vi "0_MNIST(Train).vi"() -> ()   [LabVIEW 2020]
uses:
  <vilib>/Ngene/Deep Learning Toolkit/Toolkit/NN_Train/Controls/NN_Train_Params.ctl
  <vilib>/Ngene/Deep Learning Toolkit/Toolkit/NN_Train/Controls/NN_Train_Optimizer.ctl
  <vilib>/Ngene/Deep Learning Toolkit/Toolkit/NN_Train/Controls/NN_Train_Data_Sampling.ctl
  Controls/Img_GrayScale.ctl
  <vilib>/Ngene/Deep Learning Toolkit/Toolkit/NN_Train/Controls/NN_Train_Session_Data.ctl
  <vilib>/Ngene/Deep Learning Toolkit/Toolkit/NN_Train/Controls/NN_LR_Policy_Cfg.ctl
  <vilib>/Ngene/Deep Learning Toolkit/Toolkit/NN_Train/Controls/NN_LR_Policy_Type.ctl
  <vilib>/Ngene/Deep Learning Toolkit/Toolkit/NN_Network/Controls/NN_Device.ctl
  <vilib>/Ngene/Deep Learning Toolkit/Toolkit/NN_Layers/Layers/Pool/Controls/NN_Layer_Config(Pool).ctl
  <vilib>/Ngene/Deep Learning Toolkit/Toolkit/NN_Data/API/NN_Dims(V,H).ctl
  <vilib>/Ngene/Deep Learning Toolkit/Toolkit/NN_Layers/Layers/Conv2D/Controls/NN_Conv2D_Padding_Type.ctl
  <vilib>/Ngene/Deep Learning Toolkit/Toolkit/NN_Layers/Layers/Conv2D/Controls/NN_Layer_Config(Conv2D).ctl
  <vilib>/Ngene/Deep Learning Toolkit/Toolkit/NN_Layers/Layers/Conv2D/Controls/NN_Layer_Params(Conv2D).ctl
  <vilib>/Ngene/Deep Learning Toolkit/Toolkit/NN_Layers/Layers/BatchNorm/Controls/NN_BN_Params.ctl
  <vilib>/Ngene/Deep Learning Toolkit/Toolkit/NN_Activations/Controls/NN_Activation_Type.ctl
  <vilib>/Ngene/Deep Learning Toolkit/Toolkit/NN_Layers/Controls/NN_Layer_Init_Params.ctl
  <vilib>/Ngene/Deep Learning Toolkit/Toolkit/NN_Layers/Controls/NN_Layer_Weight_Init_Type.ctl
  <vilib>/Ngene/Deep Learning Toolkit/Toolkit/NN_Layers/Layers/FC/Controls/NN_Layer_Config(FC).ctl
  <vilib>/Ngene/Deep Learning Toolkit/Toolkit/NN_Network/Controls/NN_Save_Before_Destroy_Options.ctl
  <vilib>/Ngene/Deep Learning Toolkit/Toolkit/NN_Layers/Layers/Input/Controls/NN_Layer_Config(Input3D).ctl
  <vilib>/Ngene/Deep Learning Toolkit/Toolkit/NN_Data/API/NN_Dims(C,H,W).ctl
  <vilib>/Ngene/Deep Learning Toolkit/Toolkit/NN_Data/Controls/NN_Data_type.ctl
  <vilib>/Ngene/Deep Learning Toolkit/Toolkit/NN_Layers/Layers/Input/NN_Layer_Create(Input3D).vi
  <vilib>/Ngene/Deep Learning Toolkit/Toolkit/NN_Layers/Layers/Conv2D/NN_Layer_Create(Conv2D).vi
  <vilib>/Ngene/Deep Learning Toolkit/Toolkit/NN_Layers/Layers/Pool/NN_Layer_Create(maxPool).vi
  <vilib>/Ngene/Deep Learning Toolkit/Toolkit/NN_Layers/Layers/FC/NN_Layer_Create(FC).vi
  <vilib>/Ngene/Deep Learning Toolkit/Toolkit/NN_Layers/Layers/SoftMax/NN_Layer_Create(SoftMax).vi
  <vilib>/Ngene/Deep Learning Toolkit/Toolkit/NN_Train/Loss_Functions/NN_Set_Loss(CrossEntropy).vi
  <vilib>/ptbypt/Filters.llb/FIR Filter PtByPt.vi
  <vilib>/Ngene/Deep Learning Toolkit/Toolkit/NN_Network/subVIs/NN_Predict/NN_Predict(In3D_Out1D).vi
  <vilib>/Ngene/Deep Learning Toolkit/Toolkit/NN_Train/Eval_Loss/NN_Eval_Test_Error_Loss/NN_Eval(In3D_Out1D).vi
  <vilib>/Ngene/Deep Learning Toolkit/Toolkit/NN_Train/Eval_Loss/NN_Calc_Cofusion_Matrix/NN_Calc_Confusion_Matrix(In3D_Out1D).vi
  <vilib>/Ngene/Deep Learning Toolkit/Toolkit/NN_Data/subVIs/Dataset_Destroy/NN_Datasets_All_Destroy(In3D_Out1D).vi
  <vilib>/Ngene/Deep Learning Toolkit/Toolkit/NN_Network/API/NN_Set_Input/3D/NN_Set_Input(3D_SGL_idx).vi
  <vilib>/Ngene/Deep Learning Toolkit/Toolkit/Deep_Learning_Toolkit_by_Ngene.lvlib
panel:
  in  "Tab":T1(tab)
  out "Train Speed (img/s)":dbl=1821.0660349846569 format="%#_3p"
  out "Train Graphs":T2(graph)={"Filtered x"=0.010311128, "Valid_Loss"=0.028593188, "Valid_Error"=0.0063333334}
  in  "Check_Val":bool
  out "Session Data":T3={"Epochs"=8.353684, "Tot_Iter"=3720, "LR"=0.005, "LR_iter"=3721}
  in  "Stop_Train":bool
  out "Train/Val_Metrics":T4={"Train_Loss"=0.010311128, "Valid_Loss"=0.028593188, "Valid_Error"=0.0063333334} {"Train_Loss" format="%#_4g"; "Valid_Loss" format="%#_3g"}
  in  "LR Update Policy":T5={"Policy_Type"=enum."Step", "LR0"=0.019999999998737077, "k"=4.0, "WarmUp_Policy"=enum."Step", "WarmUp_Iter"=1, "WarmUp_Ratio"=1.0} {"WarmUp_Ratio" min=1; "WarmUp_Iter" min=1; "LR0" format="%.7f"}
  out "Train Speed (s/iter)":dbl=0.07028849999998954 format="%#_2p"
  in  "Train_Params":T7={"Optimizer"=enum."Adam", "Beta_1"=0.9, "Beta_2"=0.999, "Weight Decay(L1)"=1e-07, "Weight Decay(L2)"=1e-07, "Data_Sampling"=enum."Random"}
  out "Time_Elapsed":dbl=52.864782399999996 format="%<%H:%M:%S>t"
  out "Test_Loss":sgl=0.020572739 format="%#_3g"
  out "Test_Error":sgl=0.0068
  in  "Working Dir":path=path "D:/Ngene/GitHub/deepltk_fpga_examples/1_MNIST_Classification(PXI,sbRIO)/Models/0_Original"
  in  "MNIST Dataset Path":path
  in  "NN_Device":T10=enum."GPU"
  out "Labels":string[](array[string])=["0", "1", "2", "3", "4", "5", "6", "7", "8", "9"]
  out "Draw Digit (280x280 px)":picture
  in  "Pen Color":u32(colorbox)=197379
  in  "Clear":bool
  out "Test Speed (img/s)":dbl=470.4554008281355 format="%#_2p"
  out "test time(s/img)":dbl=0.0021255999999993946 format="%#_3p"
  out "Predictions":sgl[](array[slide])=[8.9249954e-07, 0.99996126, 3.5950038e-06, 3.072444e-09, 2.722933e-09, 2.5288546e-07, 3.6905917e-07, 3.3238346e-05, 1.7368803e-12, 3.9734755e-07] scale=0.0..1.0
  in  "Pen Width":dbl=24.0
  in  "Stop Test":bool
  out "Pen Attributes":T11={"Width"=24, "Style"=enum."Solid"}
  out "image (28x28px)":sgl[][](graph)=[[-1.0, -1.0, -1.0, -1.0, -1.0, -1.0, -1.0, -1.0, -1.0, -1.0, -1.0, -1.0, -1.0, -1.0, -1.0, -1.0, -1.0, -1.0, -1.0, -1.0, -1.0, -1.0, -1.0, -1.0, -1.0, -1.0, -1.0, -1.0], [-1.0, -1.0, -1.0, -1.0, -1.0, -1.0, -1.0, -1.0, -1.0, -1.0, -1.0, -1.0, -1.0, -1.0, -1.0, -1.0, -1.0, -1.0, -1.0, -1.0, -1.0, -1.0, -1.0, -1.0, -1.0, -1.0, -1.0, -1.0], [-1.0, -1.0, -1.0, -1.0, -1.0, -1.0, -1.0, -1.0, -1.0, -1.0, -1.0, -1.0, -1.0, -1.0, -1.0, -1.0, -1.0, -1.0, -1.0, -1.0, -1.0, -1.0, -1.0, -1.0, -1.0, -1.0, -1.0, -1.0], [-1.0, -1.0, -1.0, -1.0, -1.0, -1.0, -1.0, -1.0, -1.0, -1.0, -1.0, -1.0, -1.0, -1.0, -1.0, -1.0, -1.0, -1.0, -1.0, -1.0, -1.0, -1.0, -1.0, -1.0, -1.0, -1.0, -1.0, -1.0], [-1.0, -1.0, -1.0, -1.0, -1.0, -1.0, -1.0, -1.0, -1.0, -1.0, -1.0, -1.0, -1.0, -1.0, -1.0, -1.0, -1.0, -1.0, -1.0, -1.0, -1.0, -1.0, -1.0, -1.0, -1.0, -1.0, -1.0, -1.0], [-1.0, -1.0, -1.0, -1.0, -1.0, -1.0, -1.0, -1.0, -1.0, -1.0, -1.0, -1.0, -1.0, -1.0, -1.0, -1.0, -1.0, -1.0, -1.0, -1.0, -1.0, -1.0, -1.0, -1.0, -1.0, -1.0, -1.0, -1.0], [-1.0, -1.0, -1.0, -1.0, -1.0, -1.0, -1.0, -1.0, -1.0, -1.0, -1.0, -1.0, -1.0, -1.0, -1.0, -1.0, -1.0, -1.0, -1.0, -1.0, -1.0, -1.0, -1.0, -1.0, -1.0, -1.0, -1.0, -1.0], [-1.0, -1.0, -1.0, -1.0, -1.0, -1.0, -1.0, -1.0, -1.0, -1.0, -1.0, -1.0, -1.0, -1.0, -1.0, -1.0, -1.0, -1.0, -1.0, -1.0, -1.0, -1.0, -1.0, -1.0, -1.0, -1.0, -1.0, -1.0], [-1.0, -1.0, -1.0, -1.0, -1.0, -1.0, -1.0, -1.0, -1.0, -1.0, -1.0, -1.0, -1.0, -1.0, -1.0, -1.0, -1.0, -1.0, -1.0, -1.0, -1.0, -1.0, -1.0, -1.0, -1.0, -1.0, -1.0, -1.0], [-1.0, -1.0, -1.0, -1.0, -1.0, -1.0, -1.0, -1.0, -1.0, -1.0, -1.0, -1.0, -1.0, -1.0, -1.0, -1.0, -1.0, -1.0, -1.0, -1.0, -1.0, -1.0, -1.0, -1.0, -1.0, -1.0, -1.0, -1.0], [-1.0, -1.0, -1.0, -1.0, -1.0, -1.0, -1.0, -1.0, -1.0, -1.0, -1.0, -1.0, -1.0, -1.0, -1.0, -1.0, -1.0, -1.0, -1.0, -1.0, -1.0, -1.0, -1.0, -1.0, -1.0, -1.0, -1.0, -1.0], [-1.0, -1.0, -1.0, -1.0, -1.0, -1.0, -1.0, -1.0, -1.0, -1.0, -1.0, -1.0, -1.0, -1.0, -1.0, -1.0, -1.0, -1.0, -1.0, -1.0, -1.0, -1.0, -1.0, -1.0, -1.0, -1.0, -1.0, -1.0], [-1.0, -1.0, -1.0, -1.0, -1.0, -1.0, -1.0, -1.0, -1.0, -1.0, -1.0, -1.0, -1.0, -1.0, -1.0, -1.0, -1.0, -1.0, -1.0, -1.0, -1.0, -1.0, -1.0, -1.0, -1.0, -1.0, -1.0, -1.0], [-1.0, -1.0, -1.0, -1.0, -1.0, -1.0, -1.0, -1.0, -1.0, -1.0, -1.0, -1.0, -1.0, -1.0, -1.0, -1.0, -1.0, -1.0, -1.0, -1.0, -1.0, -1.0, -1.0, -1.0, -1.0, -1.0, -1.0, -1.0], [-1.0, -1.0, -1.0, -1.0, -1.0, -1.0, -1.0, -1.0, -1.0, -1.0, -1.0, -1.0, -1.0, -1.0, -1.0, -1.0, -1.0, -1.0, -1.0, -1.0, -1.0, -1.0, -1.0, -1.0, -1.0, -1.0, -1.0, -1.0], [-1.0, -1.0, -1.0, -1.0, -1.0, -1.0, -1.0, -1.0, -1.0, -1.0, -1.0, -1.0, -1.0, -1.0, -1.0, -1.0, -1.0, -1.0, -1.0, -1.0, -1.0, -1.0, -1.0, -1.0, -1.0, -1.0, -1.0, -1.0], [-1.0, -1.0, -1.0, -1.0, -1.0, -1.0, -1.0, -1.0, -1.0, -1.0, -1.0, -1.0, -1.0, -1.0, -1.0, -1.0, -1.0, -1.0, -1.0, -1.0, -1.0, -1.0, -1.0, -1.0, -1.0, -1.0, -1.0, -1.0], [-1.0, -1.0, -1.0, -1.0, -1.0, -1.0, -1.0, -1.0, -1.0, -1.0, -1.0, -1.0, -1.0, -1.0, -1.0, -1.0, -1.0, -1.0, -1.0, -1.0, -1.0, -1.0, -1.0, -1.0, -1.0, -1.0, -1.0, -1.0], [-1.0, -1.0, -1.0, -1.0, -1.0, -1.0, -1.0, -1.0, -1.0, -1.0, -1.0, -1.0, -1.0, -1.0, -1.0, -1.0, -1.0, -1.0, -1.0, -1.0, -1.0, -1.0, -1.0, -1.0, -1.0, -1.0, -1.0, -1.0], [-1.0, -1.0, -1.0, -1.0, -1.0, -1.0, -1.0, -1.0, -1.0, -1.0, -1.0, -1.0, -1.0, -1.0, -1.0, -1.0, -1.0, -1.0, -1.0, -1.0, -1.0, -1.0, -1.0, -1.0, -1.0, -1.0, -1.0, -1.0], [-1.0, -1.0, -1.0, -1.0, -1.0, -1.0, -1.0, -1.0, -1.0, -1.0, -1.0, -1.0, -1.0, -1.0, -1.0, -1.0, -1.0, -1.0, -1.0, -1.0, -1.0, -1.0, -1.0, -1.0, -1.0, -1.0, -1.0, -1.0], [-1.0, -1.0, -1.0, -1.0, -1.0, -1.0, -1.0, -1.0, -1.0, -1.0, -1.0, -1.0, -1.0, -1.0, -1.0, -1.0, -1.0, -1.0, -1.0, -1.0, -1.0, -1.0, -1.0, -1.0, -1.0, -1.0, -1.0, -1.0], [-1.0, -1.0, -1.0, -1.0, -1.0, -1.0, -1.0, -1.0, -1.0, -1.0, -1.0, -1.0, -1.0, -1.0, -1.0, -1.0, -1.0, -1.0, -1.0, -1.0, -1.0, -1.0, -1.0, -1.0, -1.0, -1.0, -1.0, -1.0], [-1.0, -1.0, -1.0, -1.0, -1.0, -1.0, -1.0, -1.0, -1.0, -1.0, -1.0, -1.0, -1.0, -1.0, -1.0, -1.0, -1.0, -1.0, -1.0, -1.0, -1.0, -1.0, -1.0, -1.0, -1.0, -1.0, -1.0, -1.0], [-1.0, -1.0, -1.0, -1.0, -1.0, -1.0, -1.0, -1.0, -1.0, -1.0, -1.0, -1.0, -1.0, -1.0, -1.0, -1.0, -1.0, -1.0, -1.0, -1.0, -1.0, -1.0, -1.0, -1.0, -1.0, -1.0, -1.0, -1.0], [-1.0, -1.0, -1.0, -1.0, -1.0, -1.0, -1.0, -1.0, -1.0, -1.0, -1.0, -1.0, -1.0, -1.0, -1.0, -1.0, -1.0, -1.0, -1.0, -1.0, -1.0, -1.0, -1.0, -1.0, -1.0, -1.0, -1.0, -1.0], [-1.0, -1.0, -1.0, -1.0, -1.0, -1.0, -1.0, -1.0, -1.0, -1.0, -1.0, -1.0, -1.0, -1.0, -1.0, -1.0, -1.0, -1.0, -1.0, -1.0, -1.0, -1.0, -1.0, -1.0, -1.0, -1.0, -1.0, -1.0], [-1.0, -1.0, -1.0, -1.0, -1.0, -1.0, -1.0, -1.0, -1.0, -1.0, -1.0, -1.0, -1.0, -1.0, -1.0, -1.0, -1.0, -1.0, -1.0, -1.0, -1.0, -1.0, -1.0, -1.0, -1.0, -1.0, -1.0, -1.0]]
  out "Incorrectly Classified Imgs":T12[][](array[typedef])=[[{"image"=array28x28[784 elements], "Truth"=4, "Predicted"=9}, {"image"=array28x28[784 elements], "Truth"=2, "Predicted"=7}, {"image"=array28x28[784 elements], "Truth"=5, "Predicted"=3}, {"image"=array28x28[784 elements], "Truth"=9, "Predicted"=8}, {"image"=array28x28[784 elements], "Truth"=8, "Predicted"=9}, {"image"=array28x28[784 elements], "Truth"=8, "Predicted"=2}, {"image"=array28x28[784 elements], "Truth"=2, "Predicted"=1}, {"image"=array28x28[784 elements], "Truth"=5, "Predicted"=3}, {"image"=array28x28[784 elements], "Truth"=8, "Predicted"=9}, {"image"=array28x28[784 elements], "Truth"=1, "Predicted"=3}], [{"image"=array28x28[784 elements], "Truth"=6, "Predicted"=5}, {"image"=array28x28[784 elements], "Truth"=9, "Predicted"=4}, {"image"=array28x28[784 elements], "Truth"=4, "Predicted"=9}, {"image"=array28x28[784 elements], "Truth"=9, "Predicted"=5}, {"image"=array28x28[784 elements], "Truth"=7, "Predicted"=1}, {"image"=array28x28[784 elements], "Truth"=5, "Predicted"=3}, {"image"=array28x28[784 elements], "Truth"=9, "Predicted"=0}, {"image"=array28x28[784 elements], "Truth"=9, "Predicted"=3}, {"image"=array28x28[784 elements], "Truth"=5, "Predicted"=3}, {"image"=array28x28[784 elements], "Truth"=8, "Predicted"=3}], [{"image"=array28x28[784 elements], "Truth"=9, "Predicted"=4}, {"image"=array28x28[784 elements], "Truth"=5, "Predicted"=3}, {"image"=array28x28[784 elements], "Truth"=7, "Predicted"=9}, {"image"=array28x28[784 elements], "Truth"=6, "Predicted"=0}, {"image"=array28x28[784 elements], "Truth"=9, "Predicted"=8}, {"image"=array28x28[784 elements], "Truth"=4, "Predicted"=9}, {"image"=array28x28[784 elements], "Truth"=9, "Predicted"=8}, {"image"=array28x28[784 elements], "Truth"=9, "Predicted"=4}, {"image"=array28x28[784 elements], "Truth"=2, "Predicted"=4}, {"image"=array28x28[784 elements], "Truth"=5, "Predicted"=3}], [{"image"=array28x28[784 elements], "Truth"=6, "Predicted"=1}, {"image"=array28x28[784 elements], "Truth"=8, "Predicted"=0}, {"image"=array28x28[784 elements], "Truth"=3, "Predicted"=2}, {"image"=array28x28[784 elements], "Truth"=5, "Predicted"=3}, {"image"=array28x28[784 elements], "Truth"=6, "Predicted"=0}, {"image"=array28x28[784 elements], "Truth"=9, "Predicted"=7}, {"image"=array28x28[784 elements], "Truth"=1, "Predicted"=2}, {"image"=array28x28[784 elements], "Truth"=7, "Predicted"=9}, {"image"=array28x28[784 elements], "Truth"=7, "Predicted"=2}, {"image"=array28x28[784 elements], "Truth"=6, "Predicted"=0}], [{"image"=array28x28[784 elements], "Truth"=6, "Predicted"=4}, {"image"=array28x28[784 elements], "Truth"=5, "Predicted"=0}, {"image"=array28x28[784 elements], "Truth"=7, "Predicted"=1}, {"image"=array28x28[784 elements], "Truth"=5, "Predicted"=3}, {"image"=array28x28[784 elements], "Truth"=9, "Predicted"=4}, {"image"=array28x28[784 elements], "Truth"=2, "Predicted"=7}, {"image"=array28x28[784 elements], "Truth"=6, "Predicted"=8}, {"image"=array28x28[784 elements], "Truth"=3, "Predicted"=5}, {"image"=array28x28[784 elements], "Truth"=8, "Predicted"=3}, {"image"=array28x28[784 elements], "Truth"=5, "Predicted"=3}], [{"image"=array28x28[784 elements], "Truth"=3, "Predicted"=8}, {"image"=array28x28[784 elements], "Truth"=9, "Predicted"=3}, {"image"=array28x28[784 elements], "Truth"=9, "Predicted"=8}, {"image"=array28x28[784 elements], "Truth"=9, "Predicted"=8}, {"image"=array28x28[784 elements], "Truth"=9, "Predicted"=7}, {"image"=array28x28[784 elements], "Truth"=7, "Predicted"=1}, {"image"=array28x28[784 elements], "Truth"=0, "Predicted"=7}, {"image"=array28x28[784 elements], "Truth"=8, "Predicted"=2}, {"image"=array28x28[784 elements], "Truth"=2, "Predicted"=7}, {"image"=array28x28[784 elements], "Truth"=6, "Predicted"=2}], [{"image"=array28x28[784 elements], "Truth"=8, "Predicted"=6}, {"image"=array28x28[784 elements], "Truth"=7, "Predicted"=2}, {"image"=array28x28[784 elements], "Truth"=7, "Predicted"=2}, {"image"=array28x28[784 elements], "Truth"=0, "Predicted"=8}, {"image"=array28x28[784 elements], "Truth"=2, "Predicted"=7}, {"image"=array28x28[784 elements], "Truth"=5, "Predicted"=6}, {"image"=array28x28[784 elements], "Truth"=4, "Predicted"=9}, {"image"=array28x28[784 elements], "Truth"=5, "Predicted"=6}, {"image"=[], "Truth"=0, "Predicted"=0}, {"image"=[], "Truth"=0, "Predicted"=0}]]
  out "Confusion Matrix":string[][](table)=[["978", "0", "0", "0", "0", "0", "0", "1", "1", "0", "0.9980"], ["0", "1133", "1", "1", "0", "0", "0", "0", "0", "0", "0.9982"], ["0", "1", "1026", "0", "1", "0", "0", "4", "0", "0", "0.9942"], ["0", "0", "1", "1007", "0", "1", "0", "0", "1", "0", "0.9970"], ["0", "0", "0", "0", "978", "0", "0", "0", "0", "4", "0.9959"], ["1", "0", "0", "9", "0", "880", "2", "0", "0", "0", "0.9865"], ["3", "1", "1", "0", "1", "1", "950", "0", "1", "0", "0.9916"], ["0", "3", "3", "0", "0", "0", "0", "1020", "0", "2", "0.9922"], ["1", "0", "2", "2", "0", "0", "1", "0", "966", "2", "0.9918"], ["1", "0", "0", "2", "4", "1", "0", "2", "5", "994", "0.9851"], ["0.9939", "0.9956", "0.9923", "0.9863", "0.9939", "0.9966", "0.9969", "0.9932", "0.9918", "0.9920", ""]]
  out "Valid_Error":sgl=0.0063333334
  out "Valid_Loss":sgl=0.028454537
  in  "Stop_Test":bool
  # "Overview: This example demonstrates the usage of Deep Learning Toolkit for solving hand written digit recognition problem with Convolutional Neural Network (CNN).\nDataset: MNIST http://yann.lecun.com/exdb/mnist/\nRequirements: \nDeepLTK - Deep Learning Toolkit for LabVIEW (https://www.ngene.co/deep-learning-toolkit-for-labview)\nInstructions:\n1. Download MNIST dataset (4 files) from the link above and extract all files into one directory and provide the path to that directory at \"MNIST Dataset Path\" control.\n2. Set appropriate path at \"Working Dir\" control where the results of the training will be stored.\n3.  Run the VI with current configuration of the training parameters and Learning Rate update policy.\n4. Observe how the training loss is decreasing.\n5. Observe training speed.\n6. Periodically press \"Eval Validation\" button to evaluate Validation Loss/Error.\nNote that validation error evaluation influences the training speed, as the forward network inference is run for whole validation dataset."
  # "7. Hit \"Stop Train\" button when Validation Loss/Errors are not decreasing any more (~10 epochs).\n8. Observe the Test Error value - this represents the final accuracy of the trained network.\n9. Go to the Testing tab.\n10. Draw a digit in Draw Digit Interface and observe correctness of the predictions in the Predictions  indicator. Observe testing speed.\n11. Stop the VI by pressing \"Stop Test\" button on Testing tab.\n12. Go to the Incorrectly Classified Images tab and observe images that were incorrectly predicted by the network from the test dataset.\n13. Navigate to \"Confusion Matrix\" tab and observe the results on Test dataset.\n14. Observe the files generated at \"Working Dir\" directory. Navigate to Working directory. A directory with network name should have been created which should contain 3 files: model configuration file (.cfg), a file with trained weights (.bin), and a network visualization file (.svg) which can be opened in a web browser.\n15. Modify the network by changing network configuration on the block diagram. Go through the steps 3.-12. and observe influence on the test Loss/Error.\n16. (Optional) For deployment please open MNIST_Classifier(Deploy).vi.\n17. (Optional) Change \"NN_Device\" value to \"GPU\" to compare execution speeds on GPU and CPU.\n\nMore Examples:  https://github.com/ngenehub/deepltk_examples"
  # "Displaying images from the dataset that were incorrectly classified by the trained network."
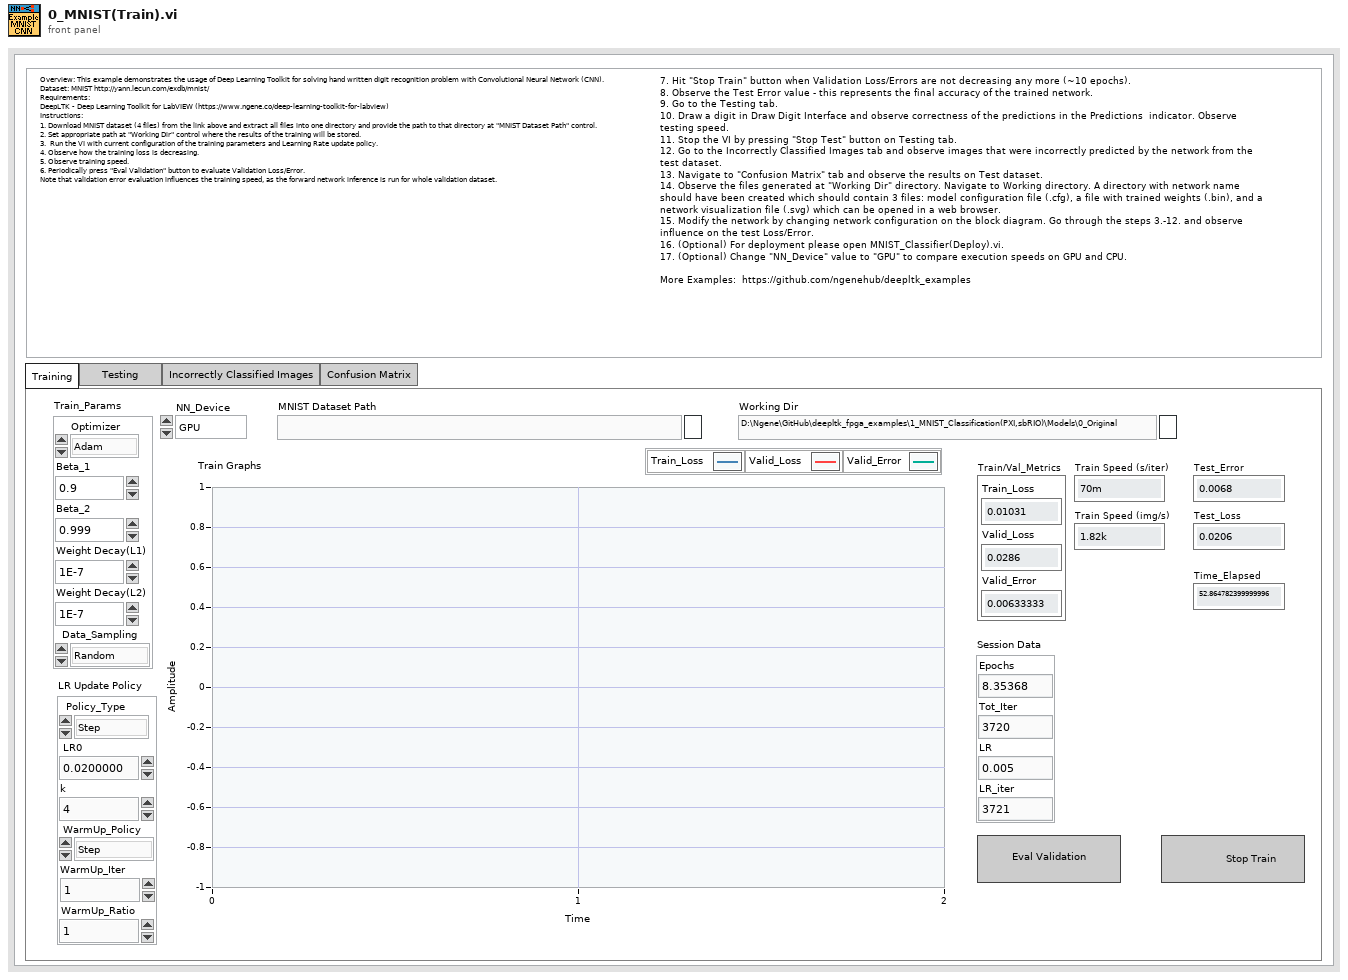
[diagram p1: front panel]
types:
  T1 = enum32{"Training", "Testing           ", "Incorrectly Classified Images", "Confusion Matrix"}
  T2 = cluster{"Filtered x":sgl, "Valid_Loss":sgl, "Valid_Error":sgl}
  T3 = typedef "Deep_Learning_Toolkit_by_Ngene.lvlib/NN_Train_Session_Data.ctl" = cluster{"Epochs":sgl, "Tot_Iter":i32, "LR":sgl, "LR_iter":i32}
  T4 = cluster{"Train_Loss":sgl, "Valid_Loss":sgl, "Valid_Error":sgl}
  T5 = typedef "Deep_Learning_Toolkit_by_Ngene.lvlib/NN_LR_Policy_Cfg.ctl" = cluster{"Policy_Type":T6, "LR0":dbl, "k":sgl, "WarmUp_Policy":enum16{"Step", "Ramp"}, "WarmUp_Iter":i32, "WarmUp_Ratio":sgl}
  T6 = typedef "Deep_Learning_Toolkit_by_Ngene.lvlib/NN_LR_Policy_Type.ctl" = enum16{"Manual", "Step", "Exp", "1/t"}
  T7 = typedef "Deep_Learning_Toolkit_by_Ngene.lvlib/NN_Train_Params.ctl" = cluster{"Optimizer":T8, "Beta_1":sgl, "Beta_2":sgl, "Weight Decay(L1)":sgl, "Weight Decay(L2)":sgl, "Data_Sampling":T9}
  T8 = typedef "Deep_Learning_Toolkit_by_Ngene.lvlib/NN_Train_Optimizer.ctl" = enum16{"SGD", "Adam", "Adagrad", "Adadelta", "RMSProp", "Nesterov"}
  T9 = typedef "Deep_Learning_Toolkit_by_Ngene.lvlib/NN_Train_Data_Sampling.ctl" = enum16{"Random", "Sequential"}
  T10 = typedef "Deep_Learning_Toolkit_by_Ngene.lvlib/NN_Device.ctl" = enum16{"CPU", "GPU"}
  T11 = cluster{"Width":u16, "Style":enum32{"Solid", "Dash", "Dot", "DashDot", "DashDotDot"}}
  T12 = typedef "Img_GrayScale.ctl" = cluster{"image":sgl[][], "Truth":i32, "Predicted":i32}
  T13 = typedef "Deep_Learning_Toolkit_by_Ngene.lvlib/NN_Layer_Config(Pool).ctl" = cluster{"Name":string, "Size":T14, "Stride":T14, "Pad_Type":T15, "Pad_Size":T14}
  T14 = typedef "Deep_Learning_Toolkit_by_Ngene.lvlib/NN_Dims(V,H).ctl" = cluster{"V":i32, "H":i32}
  T15 = typedef "Deep_Learning_Toolkit_by_Ngene.lvlib/NN_Conv2D_Padding_Type.ctl" = enum16{"Pad_Size", "Valid", "Same"}
  T16 = typedef "Deep_Learning_Toolkit_by_Ngene.lvlib/NN_Layer_Config(Conv2D).ctl" = cluster{"Name":string, "Conv_Params":T17, "BN?":bool, "BN_Params":T18, "Activation":T19, "Has Bias?":bool, "Init_Params":T20, "Custom_Params":string}
  T17 = typedef "Deep_Learning_Toolkit_by_Ngene.lvlib/NN_Layer_Params(Conv2D).ctl" = cluster{"Filters":i32, "Kernel_Size":i32, "Stride":i32, "Pad_Type":T15, "Pad_Size":i32}
  T18 = typedef "Deep_Learning_Toolkit_by_Ngene.lvlib/NN_BN_Params.ctl" = cluster{"epsilon":sgl, "momentum":sgl}
  T19 = typedef "Deep_Learning_Toolkit_by_Ngene.lvlib/NN_Activation_Type.ctl" = enum16{"Sigmoid", "ReLU", "LReLU", "ReLU6", "tanh", "Swish", "Mish", "None"}
  T20 = typedef "Deep_Learning_Toolkit_by_Ngene.lvlib/NN_Layer_Init_Params.ctl" = cluster{"Init_Type":T21, "Value":sgl}
  T21 = typedef "Deep_Learning_Toolkit_by_Ngene.lvlib/NN_Layer_Weight_Init_Type.ctl" = enum16{"Const", "Uniform", "Gaussian", "Xavier"}
  T22 = typedef "Deep_Learning_Toolkit_by_Ngene.lvlib/NN_Layer_Config(FC).ctl" = cluster{"Name":string, "Size":i32, "BN":bool, "BN_Params":T18, "Activation":T19, "Has Bias?":bool, "Init_Params":T20, "Custom_Params":string}
  T23 = typedef "Deep_Learning_Toolkit_by_Ngene.lvlib/NN_Save_Before_Destroy_Options.ctl" = cluster{"CFG?":bool, "Weights?":bool, "Render?":bool}
  T24 = typedef "Deep_Learning_Toolkit_by_Ngene.lvlib/NN_Layer_Config(Input3D).ctl" = cluster{"Name":string, "Dims":T25, "Data_Type":T26, "Shifts":sgl[], "Scales":sgl[]}
  T25 = typedef "Deep_Learning_Toolkit_by_Ngene.lvlib/NN_Dims(C,H,W).ctl" = cluster{"C":i32, "H":i32, "W":i32}
  T26 = typedef "Deep_Learning_Toolkit_by_Ngene.lvlib/NN_Data_type.ctl" = enum16{"I8", "U8", "I16", "U16", "U32 ARGB", "SGL"}
  T27 = typedef "Deep_Learning_Toolkit_by_Ngene.lvlib/NN_DataSets_All(In3D_Out1D).ctl" = cluster{"Train":T28, "Validation":T28, "Test":T28}
  T28 = typedef "Deep_Learning_Toolkit_by_Ngene.lvlib/NN_DataSet(In3D_Out1D).ctl" = cluster{"Inputs Ref.":variant, "Outputs Ref.":T29, "Dataset_Size":i32, "Dims_In":T25, "Dims_Out":i32, "Labels":string[], "File Paths":path[]}
  T29 = typedef "Deep_Learning_Toolkit_by_Ngene.lvlib/NN_Data_ref(2D_SGL).ctl" = refnum<data-value>
  T30 = typedef "Deep_Learning_Toolkit_by_Ngene.lvlib/NN.ctl" = cluster{"Name":string, "No of Layers":i32, "mBatch":i32, "Layers":T31[], "Dimty":T32, "Dims_In":T25, "Dims_Out":T25, "Working_Dir":path, "Train?":bool, "Train_Params":T7, "LR_Update_Policy":T5, "Session Data":T3, "Ground_truth":T33, "NNg_hdls":T34, "NN_Device":T10, "GPU Id":i32, "Labels":string[], "Receptive Field":T14[], "Loss_Type":T35, "Loss_Cfg_Prms":variant, "NNG_WS":T36}
  T31 = typedef "Deep_Learning_Toolkit_by_Ngene.lvlib/NN_Layer_ref.ctl" = refnum<data-value>
  T32 = typedef "Deep_Learning_Toolkit_by_Ngene.lvlib/NN_In_Out_Dim-ty.ctl" = enum8{"In1D_Out1D", "In3D_Out1D", "In3D_Out3D", "In3D_OutBBox"}
  T33 = typedef "Deep_Learning_Toolkit_by_Ngene.lvlib/NN_Ground_truth.ctl" = cluster{"Y":variant}
  T34 = typedef "Deep_Learning_Toolkit_by_Ngene.lvlib/nng_cuda_handles.ctl" = cluster{"cudnn":u64, "cublas":u64, "stream":u64, "curand":u64}
  T35 = typedef "Deep_Learning_Toolkit_by_Ngene.lvlib/NN_Loss_Type.ctl" = enum16{"None", "MSE", "CrossEntropy", "YOLO_v2", "YOLO_v4"}
  T36 = typedef "Deep_Learning_Toolkit_by_Ngene.lvlib/NNG_WS.ctl" = cluster{"NNG_WS_Mem":T37, "Max_WS_Size":i64}
  T37 = typedef "Deep_Learning_Toolkit_by_Ngene.lvlib/NNg_WS_Mem_DVR.ctl" = refnum<data-value>
  T38 = typedef "Deep_Learning_Toolkit_by_Ngene.lvlib/NN_Eval_Params.ctl" = cluster{"Loss":sgl, "Error":sgl}
  T39 = typedef "Deep_Learning_Toolkit_by_Ngene.lvlib/NN_Layer.ctl" = cluster{"Name":string, "Layer_Data":variant, "Layer_Type":T40, "Dims_In":T25, "Layers_In":variant, "Dims_Out":T25, "Layers_Out":variant, "Metrics":T41, "GPU_Data":variant, "mBatch":i32, "NN_Device":T10, "NNg_hdls":T34, "Train?":bool, "Dimty":T42, "RecptField":T43}
  T40 = typedef "Deep_Learning_Toolkit_by_Ngene.lvlib/NN_Layer_Type.ctl" = enum16{"Input1D", "Input3D", "Conv1D", "Conv2D", "Conv2D_Adv", "MaxPool", "AvgPool", "UpSample", "DropOut3D", "ShortCut", "Concat", "SoftMax3D", "FC", "DropOut", "Softmax", "Flatten", "YOLO_v2", "YOLO_v4", "Activation", "BatchNormalization", "Unsupported"}
  T41 = typedef "Deep_Learning_Toolkit_by_Ngene.lvlib/NN_Layer_Metrics.ctl" = cluster{"Data":dbl, "Params":dbl, "Ops":dbl}
  T42 = typedef "Deep_Learning_Toolkit_by_Ngene.lvlib/NN_Layer_Dimty.ctl" = enum16{"1D", "3D"}
  T43 = typedef "Deep_Learning_Toolkit_by_Ngene.lvlib/NN_Layer_RF_State.ctl" = cluster{"Dims":T14, "J":T14}
  T44 = cluster{"left":i16, "top":i16, "right":i16, "bottom":i16}
  T45 = typedef "LVMouseTypeDef.ctl" = cluster{"Mouse Position":cluster{"X":i32, "Y":i32}, "Mouse Modifiers":cluster{"Button Down":bool, "Shift Mod":bool, "Menu Mod":bool, "Option Mod":bool}}
  T46 = typedef "imagedata.ctl" = cluster{"image type":i32, "image depth":i32, "image":u8[], "mask":u8[], "colors":u32[], "Rectangle":cluster{"left":i16, "top":i16, "right":i16, "bottom":i16}}
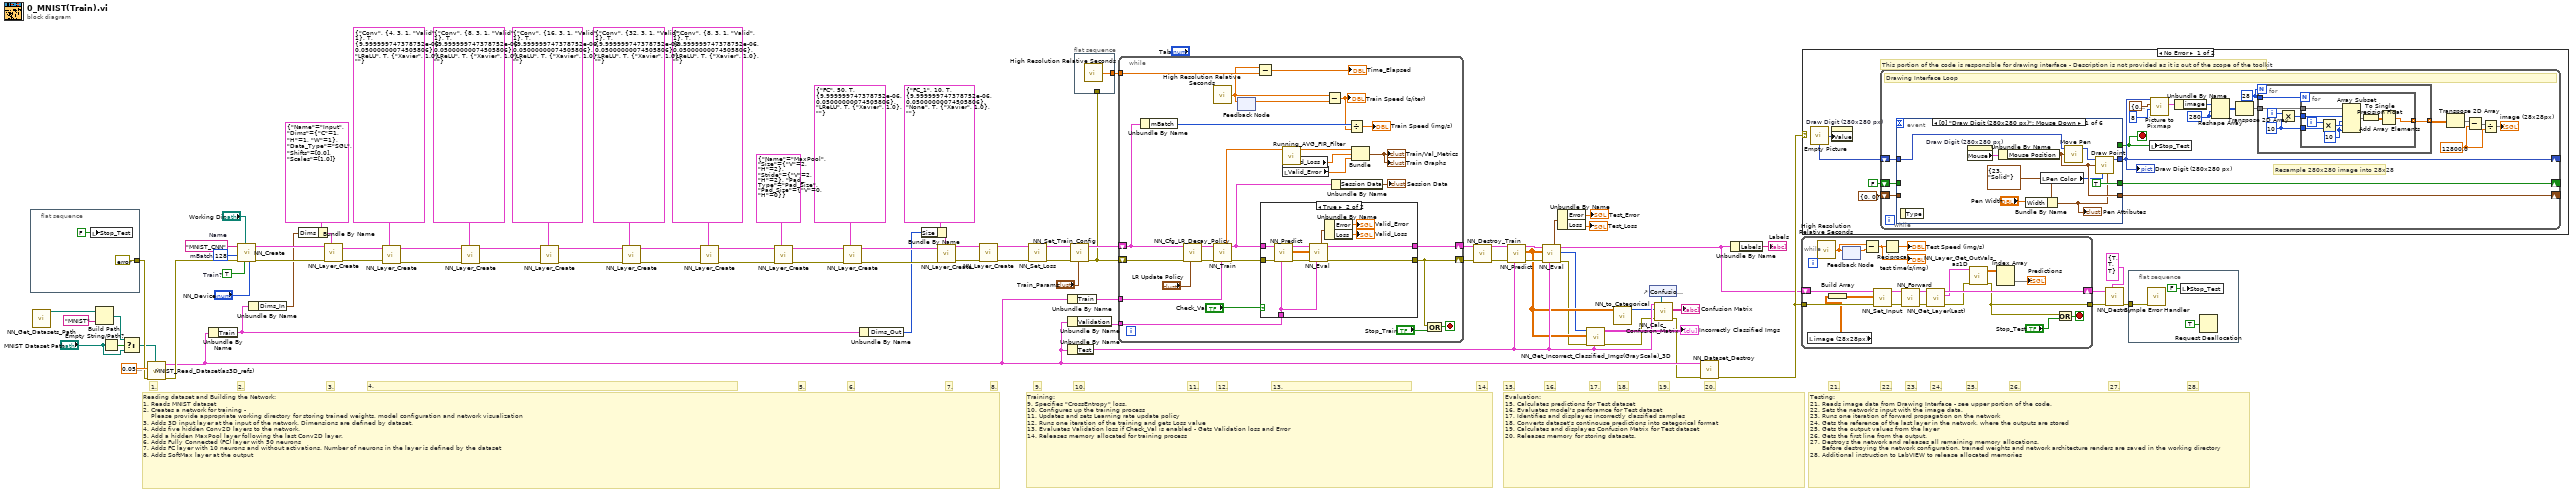
[diagram p0: block diagram]
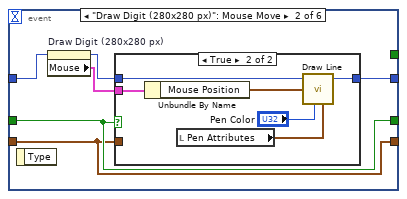
[diagram p3: hidden frame]
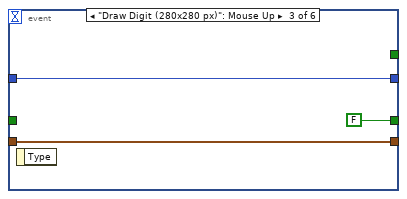
[diagram p5: hidden frame]
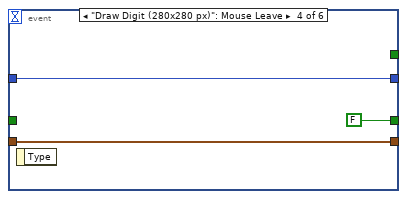
[diagram p6: hidden frame]
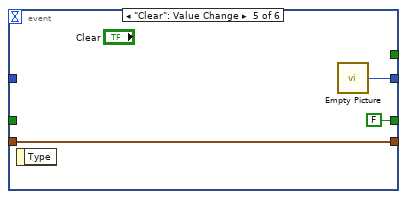
[diagram p7: hidden frame]
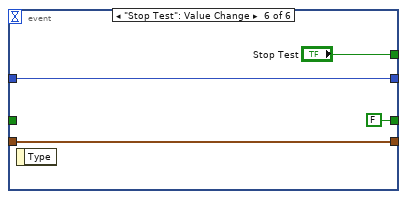
[diagram p8: hidden frame]
diagram:
  w64 = TRUE  # Train?
  w76 = 128  # mBatch
  w84 = "MNIST_CNN"  # Name
  # "28."
  # "27."
  # "Evaluation:\n15. Calculates predictions for Test dataset\n16. Evaluates model's perforamce for Test dataset\n17. Identifies and displayes incorrectly classified samples\n18. Converts dataset's continouse predictions into categorical format\n19. Calculates and displayes Confusion Matrix for Test dataset\n20. Releases memory for storing datasets."
  # "18."
  # "16."
  # "26."
  # "25."
  # "Testing:\n21. Reads image data from Drawing Interface - see upper portion of the code.\n22. Sets the network's input with the image data.\n23. Runs one iteration of forward propagation on the network\n24. Gets the reference of the last layer in the network, where the outputs are stored\n25. Gets the output values from the layer\n26. Gets the first line from the output.\n27. Destroys the network and releases all remaining memory allocations.\n      Before destroying the network configuration, trained weights and network architecture renders are saved in the working directory\n28. Additional instruction to LabVIEW to release allocated memories"
  # "24."
  # "Training:\n9. Specifies \"CrossEntropy\" loss.\n10. Configures up the training process\n11. Updates and sets Learning rate update policy\n12. Runs one iteration of the training and gets Loss value\n13. Evaluates Validation loss if Check_Val is enabled - Gets Validation loss and Error\n14. Releases memory allocated for training process"
  # "Reading dataset and Building the Network:\n1.\tReads MNIST dataset\n2.\tCreates a network for training -\n    Please provide appropriate working directory for storing trained weights, model configuration and network visualization\n3.\tAdds 3D input layer at the input of the network. Dimensions are defined by dataset.\n4.\tAdds five hidden Conv2D layers to the network.\n5.\tAdd a hidden MaxPool layer following the last Conv2D layer.\n6.\tAdds Fully Connected (FC) layer with 50 neurons\n7.\tAdds FC layer with 10 neurons and without activations. Number of neurons in the layer is defined by the dataset\n8.\tAdds SoftMax layer at the output"
  # "23."
  # "22."
  # "21."
  # "20."
  # "19."
  # "17."
  # "15."
  # "14."
  # "13."
  # "12."
  # "11."
  # "10."
  # "9."
  # "8."
  # "7."
  # "6."
  # "5."
  # "4."
  # "3."
  # "2."
  # "1."
  n1 = flat-sequence {
    tunnel: [errorcluster {"status"=FALSE, "code"=0, "source"=""} ("error in (no error)")] -> w68
    frame #0 {
      n2 = local write "Stop_Test"(FALSE ("Stop_Test")) -> ()
    }
  }
  n3 = call "NN_Get_Datasets_Path.vi"() -> ("Datasets path"=w1:path)  [unwired: 11 in]
  n4 = Build Path(base path=w1, name or relative path="MNIST") -> (appended path=w5:path)
  n5 = Empty String/Path?(string/path="MNIST Dataset Path") -> (empty?=w4:bool)
  n6 = Select(t=w5, s=w4, f="MNIST Dataset Path") -> (s? t:f=w2:path)
  n7 = call "MNIST_Read_Dataset(as3D_refs).vi"("MNIST Dataset Path"=w2, "error in"=w68, "Validation_Size"=sgl 0.05 ("Valid_data_Size")) -> ("error out"=w85:errorcluster, "Data(3D)_Refs"=w47:T27)  [unwired: 7 in]
  n8 = Unbundle By Name(w47) -> ("Train"=w46:T28)
  n9 = call <vilib>:"NN_Create.vi"("NN_Device"="NN_Device", "Train? (false)"=w64, "Working Dir"="Working Dir", "error in (no error)"=w85, "mBatch (1)"=w76, "Name"=w84) -> ("error out"=w82:errorcluster, "NN out"=w83:T30)  [unwired: 4 in]
  n10 = Unbundle By Name(w46) -> ("Dims_In"=w48:T25)
  n11 = Bundle By Name(cluster=T24 {"Name"="Input", "Dims"={"C"=1, "H"=1, "W"=1}, "Data_Type"=enum."SGL", "Shifts"=[0.0], "Scales"=[1.0]} ("Cluster"), "Dims"=w48) -> (w69:T24)
  n12 = call-poly <vilib>:"NN_Layer_Create.vi"("Input3D_Cfg"=w69, "error in (no error)"=w82, "NN In"=w83) -> ("error out"=w57:errorcluster, "NN out"=w34:T30)  [unwired: 6 in, 1 out]
  n13 = call-poly <vilib>:"NN_Layer_Create.vi"("Conv2D_Cfg"=T16 {"Name"="Conv", "Conv_Params"={"Filters"=4, "Kernel_Size"=3, "Stride"=1, "Pad_Type"=enum."Valid", "Pad_Size"=1}, "BN?"=TRUE, "BN_Params"={"epsilon"=1e-05, "momentum"=0.05}, "Activation"=enum."LReLU", "Has Bias?"=TRUE, "Init_Params"={"Init_Type"=enum."Xavier", "Value"=1.0}, "Custom_Params"=""} ("Layer_Config_Params"), "error in (no error)"=w57, "NN in"=w34) -> ("error out"=w19:errorcluster, "NN out"=w20:T30)  [unwired: 6 in, 1 out]
  n14 = call-poly <vilib>:"NN_Layer_Create.vi"("Conv2D_Cfg"=T16 {"Name"="Conv", "Conv_Params"={"Filters"=8, "Kernel_Size"=3, "Stride"=1, "Pad_Type"=enum."Valid", "Pad_Size"=1}, "BN?"=TRUE, "BN_Params"={"epsilon"=1e-05, "momentum"=0.05}, "Activation"=enum."LReLU", "Has Bias?"=TRUE, "Init_Params"={"Init_Type"=enum."Xavier", "Value"=1.0}, "Custom_Params"=""} ("Layer_Config_Params"), "error in (no error)"=w19, "NN in"=w20) -> ("error out"=w16:errorcluster, "NN out"=w17:T30)  [unwired: 6 in, 1 out]
  n15 = call-poly <vilib>:"NN_Layer_Create.vi"("Conv2D_Cfg"=T16 {"Name"="Conv", "Conv_Params"={"Filters"=16, "Kernel_Size"=3, "Stride"=1, "Pad_Type"=enum."Valid", "Pad_Size"=1}, "BN?"=TRUE, "BN_Params"={"epsilon"=1e-05, "momentum"=0.05}, "Activation"=enum."LReLU", "Has Bias?"=TRUE, "Init_Params"={"Init_Type"=enum."Xavier", "Value"=1.0}, "Custom_Params"=""} ("Layer_Config_Params"), "error in (no error)"=w16, "NN in"=w17) -> ("error out"=w13:errorcluster, "NN out"=w14:T30)  [unwired: 6 in, 1 out]
  n16 = call-poly <vilib>:"NN_Layer_Create.vi"("Conv2D_Cfg"=T16 {"Name"="Conv", "Conv_Params"={"Filters"=32, "Kernel_Size"=3, "Stride"=1, "Pad_Type"=enum."Valid", "Pad_Size"=1}, "BN?"=TRUE, "BN_Params"={"epsilon"=1e-05, "momentum"=0.05}, "Activation"=enum."LReLU", "Has Bias?"=TRUE, "Init_Params"={"Init_Type"=enum."Xavier", "Value"=1.0}, "Custom_Params"=""} ("Layer_Config_Params"), "error in (no error)"=w13, "NN in"=w14) -> ("error out"=w10:errorcluster, "NN out"=w11:T30)  [unwired: 6 in, 1 out]
  n17 = call-poly <vilib>:"NN_Layer_Create.vi"("Conv2D_Cfg"=T16 {"Name"="Conv", "Conv_Params"={"Filters"=8, "Kernel_Size"=3, "Stride"=1, "Pad_Type"=enum."Valid", "Pad_Size"=1}, "BN?"=TRUE, "BN_Params"={"epsilon"=1e-05, "momentum"=0.05}, "Activation"=enum."LReLU", "Has Bias?"=TRUE, "Init_Params"={"Init_Type"=enum."Xavier", "Value"=1.0}, "Custom_Params"=""} ("Layer_Config_Params"), "error in (no error)"=w10, "NN in"=w11) -> ("error out"=w8:errorcluster, "NN out"=w9:T30)  [unwired: 6 in, 1 out]
  n18 = call-poly <vilib>:"NN_Layer_Create.vi"("MaxPool_Cfg"=T13 {"Name"="MaxPool", "Size"={"V"=2, "H"=2}, "Stride"={"V"=2, "H"=2}, "Pad_Type"=enum."Pad_Size", "Pad_Size"={"V"=0, "H"=0}}, "error in (no error)"=w8, "NN in"=w9) -> ("error out"=w53:errorcluster, "NN out"=w55:T30)  [unwired: 6 in, 1 out]
  n19 = call-poly <vilib>:"NN_Layer_Create.vi"("FC_Cfg"=T22 {"Name"="FC", "Size"=50, "BN"=TRUE, "BN_Params"={"epsilon"=1e-05, "momentum"=0.05}, "Activation"=enum."LReLU", "Has Bias?"=TRUE, "Init_Params"={"Init_Type"=enum."Xavier", "Value"=1.0}, "Custom_Params"=""} ("Layer_Config_Params"), "error in (no error)"=w53, "NN in"=w55) -> ("error out"=w59:errorcluster, "NN out"=w58:T30)  [unwired: 6 in, 1 out]
  n20 = Unbundle By Name(w46) -> ("Dims_Out"=w45:i32)
  n21 = Bundle By Name(cluster=T22 {"Name"="FC_1", "Size"=10, "BN"=TRUE, "BN_Params"={"epsilon"=1e-05, "momentum"=0.05}, "Activation"=enum."None", "Has Bias?"=TRUE, "Init_Params"={"Init_Type"=enum."Xavier", "Value"=1.0}, "Custom_Params"=""} ("Layer_Config_Params"), "Size"=w45) -> (w56:T22)
  n22 = call-poly <vilib>:"NN_Layer_Create.vi"("FC_Cfg"=w56, "error in (no error)"=w59, "NN in"=w58) -> ("error out"=w72:errorcluster, "NN out"=w73:T30)  [unwired: 6 in, 1 out]
  n23 = call-poly <vilib>:"NN_Layer_Create.vi"("error in (no error)"=w72, "NN in"=w73) -> ("error out"=w51:errorcluster, "NN out"=w54:T30)  [unwired: 7 in, 1 out]
  n24 = call-poly <vilib>:"NN_Set_Loss.vi"("error in (no error)"=w51, "NN in"=w54) -> ("error out"=w50:errorcluster, "NN out"=w52:T30)  [unwired: 8 in]
  n25 = Unbundle By Name(w47) -> ("Train"=w49:T28)
  n26 = Unbundle By Name(w47) -> ("Validation"=w75:T28)
  n27 = Unbundle By Name(w47) -> ("Test"=w36:T28)
  n28 = call <vilib>:"NN_Set_Train_Config.vi"("NN_Train_Params"="Train_Params", "error in (no error)"=w50, "NN in"=w52) -> ("error out"=w65:errorcluster, "NN out"=w66:T30)  [unwired: 7 in]
  n29 = flat-sequence {
    tunnel: [w88] -> w78
    tunnel: w65 -> [_]
    frame #0 {
      n30 = call <vilib>:"High Resolution Relative Seconds.vi"() -> ("relative seconds"=w88:dbl)
    }
  }
  n31 = while {
    shift-right: [w96] -> w41
    shift-left: w65 -> [w90]
    shift-right: [w93] -> w42
    shift-left: w66 -> [w91]
    tunnel: w78 -> [w105]
    tunnel: w49 -> [w95]
    tunnel: w75 -> [w89]
    stop <- w113 stop-if-true
    n32 = Unbundle By Name(w91) -> ("mBatch"=w101:i32)
    n33 = call <vilib>:"NN_Cfg_LR_Decay_Policy.vi"("LR_Decay_Params"="LR Update Policy", "error in (no error)"=w90, "NN in"=w91) -> ("error out"=w108:errorcluster, "NN out"=w114:T30)  [unwired: 7 in]
    n34 = call <vilib>:"High Resolution Relative Seconds.vi"() -> ("relative seconds"=w104:dbl)
    n35 = call <vilib>:"NN_Train.vi"("Train Dataset"=w95, "error in (no error)"=w108, "NN in"=w114) -> ("error out"=w97:errorcluster, "NN out"=w92:T30, "Loss"=w109:sgl)  [unwired: 3 in, 3 out]
    n36 = feedback #1() -> (w115:dbl)  [unwired: 1 in]
    n37 = feedback-in #1(w104) -> ()
    n38 = Subtract(x=w104, y=w105) -> (x-y=→"Time_Elapsed":dbl)
    n39 = case shown="True" "Check_Val" {
      tunnel: w92 -> [w116 w128]
      tunnel: w97 -> [w117 w124]
      tunnel: [w117 w126] -> w96
      tunnel: [w116 w127] -> w93
      tunnel: w89 -> [_ w121]
      frame False {
      }
      frame True {
        n40 = call-poly <vilib>:"NN_Predict.vi"("Dataset"=w121, "error in (no error)"=w124, "NN in"=w128) -> ("error out"=w123:errorcluster, "Predictions"=w122:sgl[][], "NN out"=w125:T30)  [unwired: 6 in]
        n41 = call-poly <vilib>:"NN_Eval.vi"("Dataset"=w121, "error in (no error)"=w123, "Predictions"=w122, "NN in"=w125) -> ("error out"=w126:errorcluster, "NN out"=w127:T30, "NN_Eval_Params"=w120:T38)  [unwired: 4 in, 1 out]
        n42 = Unbundle By Name(w120) -> ("Error"=→"Valid_Error":sgl, "Loss"=→"Valid_Loss":sgl)
      }
    }
    n43 = call <vilib>:"Running_AVG_FIR_Filter.vi"("Numeric"=w109) -> ("Filtered x"=w110:sgl)  [unwired: 10 in]
    n44 = local read "Valid_Loss"() -> (w112:sgl)
    n45 = local read "Valid_Error"() -> (w107:sgl)
    n46 = Subtract(x=w104, y=w115) -> (x-y=w99:dbl)
    "Train Speed (s/iter)" <- w99
    n47 = Unbundle By Name(w92) -> ("Session Data"=→"Session Data":T3)
    n48 = Divide(x=w101, y=w99) -> (x/y=→"Train Speed (img/s)":dbl)
    n49 = Bundle("Filtered x"=w110, "Valid_Loss"=w112, "Valid_Error"=w107) -> (→"Train Graphs" →"Train/Val_Metrics":T2)  [unwired: 1 in]
    n50 = Compound Arithmetic op=OR(w96, "Stop_Train") -> (w113:bool)
  }
  n51 = call <vilib>:"NN_Destroy_Train.vi"("error in (no error)"=w41, "NN in"=w42) -> ("error out"=w38:errorcluster, "NN out"=w40:T30)  [unwired: 8 in]
  n52 = call-poly <vilib>:"NN_Predict.vi"("Dataset"=w36, "error in (no error)"=w38, "NN in"=w40) -> ("error out"=w37:errorcluster, "Predictions"=w32:sgl[][], "NN out"=w39:T30)  [unwired: 6 in]
  n53 = call-poly <vilib>:"NN_Eval.vi"("Dataset"=w36, "error in (no error)"=w37, "Predictions"=w32, "NN in"=w39) -> ("error out"=w29:errorcluster, "Incrct_Class_idx"=w25:i32[], "NN out"=w31:T30, "NN_Eval_Params"=w22:T38)  [unwired: 4 in]
  n54 = Unbundle By Name(w22) -> ("Error"=→"Test_Error":sgl, "Loss"=→"Test_Loss":sgl)
  n55 = call "NN_Get_Incorrect_Classified_Imgs(GrayScale)_3D.vi"("Test_Data"=w36, "error in (no error)"=w29, "Predictions"=w32, "MisClassed_idx"=w25) -> ("error out"=w28:errorcluster, "Images(GrayScale)"=→"Incorrectly Classified Imgs":T12[][])  [unwired: 6 in]
  n56 = call <vilib>:"NN_to_Categorical.vi"("Prediction"=w32) -> ("Label_Idx"=w33:i32[])  [unwired: 10 in]
  n57 = control-ref of="Confusion Matrix"() -> (w43:refnum<vi>)
  n58 = call-poly <vilib>:"NN_Calc_Confusion_Matrix.vi"("Confusion Matrix (Table) ref."=w43, "error in (no error)"=w28, "Predictions"=w33, "Dataset"=w36) -> ("error out"=w27:errorcluster, "Confusion Matrix (Table)"=→"Confusion Matrix":string[][])  [unwired: 3 in, 3 out]
  n59 = call-poly <vilib>:"NN_Dataset_Destroy.vi"("error in (no error)"=w27, "Datasets_All(In3D_Out1D)"=w47) -> ("error out"=w67:errorcluster)  [unwired: 9 in]
  n60 = Unbundle By Name(w31) -> ("Labels"=→"Labels":string[])
  n61 = while {
    shift-right: [w147] -> w80
    shift-left: w31 -> [w140]
    tunnel: w67 -> [w138]
    tunnel: [w130] -> w79
    stop <- w145 stop-if-true
    n62 = local read "image (28x28px)"() -> (w136:sgl[][])
    n63 = call <vilib>:"High Resolution Relative Seconds.vi"() -> ("relative seconds"=w143:dbl)
    n64 = Build Array(w136) -> (w129:sgl[][][])
    n65 = feedback #2() -> (w144:dbl)  [unwired: 1 in]
    n66 = feedback-in #2(w143) -> ()
    n67 = Subtract(x=w143, y=w144) -> (x-y=w142:dbl)
    "test time(s/img)" <- w142
    n68 = call-poly <vilib>:"NN_Set_Input.vi"("error in (no error)"=w138, "Data_In(3D_SGL)"=w129, "NN in"=w140) -> ("error out"=w137:errorcluster, "NN out"=w139:T30)  [unwired: 7 in]
    n69 = Reciprocal(x=w142) -> (1/x=→"Test Speed (img/s)":dbl)
    n70 = call <vilib>:"NN_Forward.vi"("error in (no error)"=w137, "NN in"=w139) -> ("error out"=w146:errorcluster, "NN out"=w148:T30)  [unwired: 6 in, 2 out]
    n71 = call <vilib>:"NN_Get_Layer(Last).vi"("error in (no error)"=w146, "NN in"=w148) -> ("error out"=w131:errorcluster, "Last_Layer"=w135:T39, "NN out"=w147:T30)  [unwired: 6 in, 1 out]
    n72 = call <vilib>:"NN_Layer_Get_OutVals_as1D.vi"("error in (no error)"=w131, "Layer"=w135) -> ("error out"=w130:errorcluster, "Out(as1D)"=w134:sgl[][])  [unwired: 8 in]
    n73 = Index Array(array=w134) -> (element=→"Predictions":sgl[])  [unwired: 2 in]
    n74 = Or(x=w130, y="Stop_Test") -> (x .or. y?=w145:bool)
  }
  n75 = case shown="No Error" w67 {
    frame No Error {
      # "This portion of the code is responsible for drawing interface - Description is not provided as it is out of the scope of the toolkit"
      n76 = call "Empty Picture"() -> ("empty picture"=w151:picture)
      n77 = property on="Draw Digit (280x280 px)" class="Pict"("Value"=w151) -> ()  [unwired: 2 in, 2 out]
      n78 = while {
        shift-right: [w166] -> _
        shift-left: w151 -> [w171]
        shift-right: [w169] -> _
        shift-left: FALSE -> [w170]
        shift-right: [w167] -> _
        shift-left: cluster{"X":i32, "Y":i32} {"X"=0, "Y"=0} ("Mouse Position") -> [w168]
        stop <- w156 stop-if-true
        w153 = sgl 12800.0 ("dimension size")
        w157 = 280 ("dimension size")
        w159 = 28
        # "Resample 280x280 image into 28x28"
        # "Drawing Interface Loop"
        n79 = event shown="[0] \"Draw Digit (280x280 px)\": Mouse Down" {
          selector: _ -> [_ _ _ _ _ _]
          dyn-events: _ -> [_ _ _ _ _ _]
          timeout: _ -> [_ _ _ _ _ _]
          tunnel: [_ _ _ _ _ "Stop Test"] -> w156
          tunnel: [w193 w200 w211 w214 w217 w220] -> w166
          tunnel: w171 -> [w195 w199 w211 w214 _ w220]
          tunnel: w170 -> [_ w198 _ _ _ _]
          tunnel: [TRUE w198 FALSE FALSE FALSE FALSE] -> w169
          tunnel: w168 -> [_ w197 w209 w213 w216 w219]
          tunnel: [w191 w197 w209 w213 w216 w219] -> w167
          event "Draw Digit (280x280 px)": Mouse Down {
            # "Set the pen position, and draw an initial point or line."
            n80 = event-data() -> ()  [unwired: 1 in, 1 out]
            n81 = property on="Draw Digit (280x280 px)" class="Pict"() -> ("Mouse"=w196:T45)  [unwired: 2 in, 2 out]
            n82 = Unbundle By Name(w196) -> ("Mouse Position"=w191:cluster{"X":i32, "Y":i32})
            n83 = Bundle By Name(cluster=T11 {"Width"=23, "Style"=enum."Solid"} ("Pen Attributes"), "Width"="Pen Width") -> (w187:T11)
            "Pen Attributes" <- w187
            n84 = local read "Pen Color"() -> (w190:u32)
            n85 = call <vilib>:"Move Pen.vi"("new position"=w191, "picture"=w195) -> ("new picture"=w194:picture)  [unwired: 3 in]
            n86 = call <vilib>:"Draw Point.vi"("picture"=w194, "point(x,y)"=w191, "color(black)"=w190, "pen"=w187) -> ("new picture"=w193:picture)  [unwired: 5 in]
          }
          event "Draw Digit (280x280 px)": Mouse Move {
            # "Only draw if a Mouse Down event has occurred, but not a Mouse Up. Then, determine if the user is Drawing a point, a line, or selecting a subset and perform those operations in the case structure."
            n87 = event-data() -> ()  [unwired: 1 in, 1 out]
            n88 = property on="Draw Digit (280x280 px)" class="Pict"() -> ("Mouse"=w201:T45)  [unwired: 2 in, 2 out]
            n89 = case shown="True" w198 {
              tunnel: w199 -> [w202 w208]
              tunnel: w201 -> [_ w207]
              tunnel: [w202 w205] -> w200
              tunnel: w197 -> [_ _]
              frame False {
              }
              frame True {
                n90 = Unbundle By Name(w207) -> ("Mouse Position"=w206:cluster{"X":i32, "Y":i32})
                n91 = local read "Pen Attributes"() -> (w204:T11)
                n92 = call <vilib>:"Draw Line.vi"("picture"=w208, "end point"=w206, "color(black)"="Pen Color", "pen"=w204) -> ("new picture"=w205:picture)  [unwired: 5 in]
              }
            }
          }
          event "Draw Digit (280x280 px)": Mouse Up {
            # "When the user is finished drawing, we complete the operation. The only operation that we need to complete the Select Subset operation."
            n93 = event-data() -> ()  [unwired: 1 in, 1 out]
          }
          event "Draw Digit (280x280 px)": Mouse Leave {
            # "Change to the default cursor when the mouse leaves the picture."
            n94 = event-data() -> ()  [unwired: 1 in, 1 out]
          }
          event "Clear": Value Change {
            # "Erase the picture."
            n95 = event-data() -> ()  [unwired: 1 in, 1 out]
            n96 = call "Empty Picture"() -> ("empty picture"=w217:picture)
          }
          event "Stop Test": Value Change {
            # "Stop the VI."
            n97 = event-data() -> ()  [unwired: 1 in, 1 out]
          }
        }
        "Draw Digit (280x280 px)" <- w166
        n98 = local write "Stop_Test"(w156) -> ()
        n99 = call <vilib>:"Picture to Pixmap.vi"("depth"=8, "rect"=T44 {"left"=0, "top"=0, "right"=280, "bottom"=280}, "picture"=w166) -> ("image data"=w164:T46)  [unwired: 7 in, 1 out]
        n100 = Unbundle By Name(w164) -> ("image"=w162:u8[])
        n101 = Reshape Array(w162, w157, w157) -> (w161:u8[][])
        n102 = Transpose 2D Array(2D array=w161) -> (transposed array=w160:u8[][])
        n103 = for {
          N: w159 -> [_]
          tunnel: w160 -> [w177]
          tunnel: w159 -> [w176]
          tunnel: [w172] -> w158 mode=indexing
          i -> [w175]
          w173 = 10 ("x")
          n104 = Multiply(x=w175, y=w173) -> (x*y=w174:i32)
          n105 = for {
            N: w176 -> [_]
            tunnel: w177 -> [w186]
            tunnel: w174 -> [w185]
            tunnel: w173 -> [w182]
            tunnel: [w178] -> w172 mode=indexing
            i -> [w184]
            w181 = 10 ("length")
            n106 = Multiply(x=w184, y=w182) -> (x*y=w183:i32)
            n107 = Array Subset(array=w186, index (row)=w185, length (row)=w181, index (col)=w183, length (col)=w181) -> (w180:u8[][])
            n108 = To Single Precision Float(number=w180) -> (single precision float=w179:sgl[][])
            n109 = Add Array Elements(numeric array=w179) -> (sum=w178:sgl)
          }
        }
        n110 = Transpose 2D Array(2D array=w158) -> (transposed array=w154:sgl[][])
        n111 = Subtract(x=w154, y=w153) -> (x-y=w155:sgl[][])
        n112 = Divide(x=w155, y=w153) -> (x/y=→"image (28x28px)":sgl[][])
      }
    }
    frame Error {
    }
  }
  n113 = call <vilib>:"NN_Destroy.vi"("Save (T, T, T)"=T23 {"CFG?"=TRUE, "Weights?"=TRUE, "Render?"=TRUE} ("Save_Config"), "error in (no error)"=w79, "NN in"=w80) -> ("error out"=w81:errorcluster)  [unwired: 7 in, 1 out]
  n114 = flat-sequence {
    tunnel: w81 -> [w223]
    frame #0 {
      n115 = call <vilib>:"Simple Error Handler.vi"("error in (no error)"=w223) -> ()  [unwired: 4 in, 5 out]
      n116 = local write "Stop_Test"(FALSE ("Stop_Test")) -> ()
      n117 = Request Deallocation(TRUE ("flag")) -> ()
    }
  }
